vi "Initialize - NI.vi"(8 "error in (no error)":errorcluster, 9 "Reset":bool=TRUE, 10 "ID Query":bool=TRUE, 11 "Instrument Descriptor":refnum<k15>="Dev1") -> (0 "error out":errorcluster, 3 "instrument handle out":refnum<k15>)   [LabVIEW 2020]
panel:
  # "Do Query"
  # "Reset Device"
  # "Skip Query"
  # "Don't Reset"
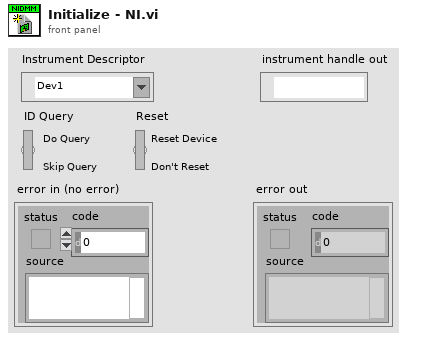
[diagram p1: front panel]
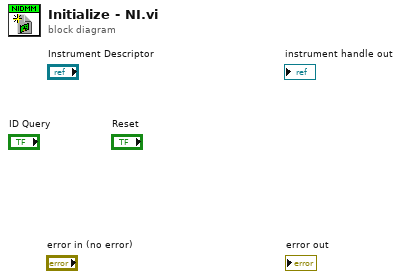
[diagram p0: block diagram]
diagram:
